vi "Read Lifetime.vi"(11 "Actor in":refnum<class "Actor.lvclass">) -> (2 "Lifetime":T1=enum."Setup")   [LabVIEW 2020, in "jettl.lvlib" / "Actor.lvclass"]
uses:
  Actor.lvclass
  Lifetime.ctl
  jettl.lvlib
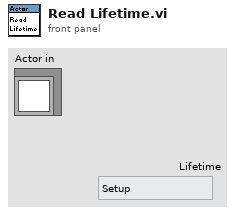
[diagram p1: front panel]
types:
  T1 = typedef "jettl.lvlib/Lifetime.ctl" = enum16{"Init", "Spawn", "Setup", "Teardown Before Started", "Start", "Started", "Stopping With Children", "Stopping Without Children", "Teardown After Started", "Stopped"}
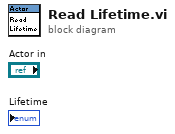
[diagram p0: block diagram]
diagram:
